vi "SUB_ContinueCom1Read.vi"(3 "error out 2":errorcluster, 4 "Numeric":i32, 5 "duplicate VISA resource name 2":refnum<visa-resource-name>) -> (0 "error out":errorcluster, 1 "String":string, 2 "duplicate VISA resource name":refnum<visa-resource-name>)   [LabVIEW 2011]
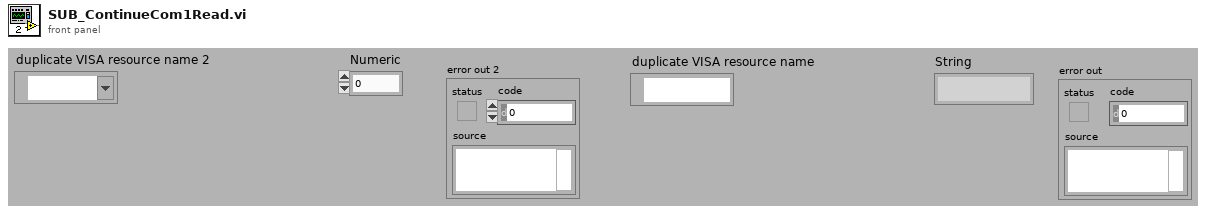
[diagram p1: front panel]
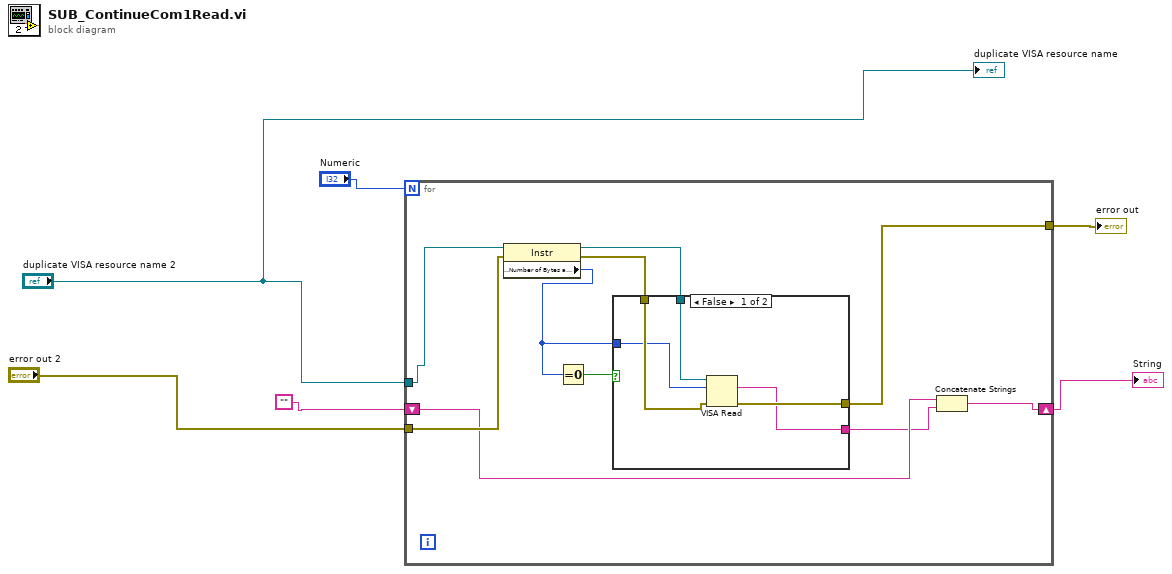
[diagram p0: block diagram]
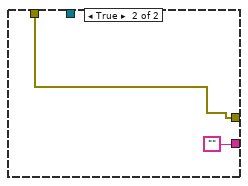
[diagram p2: hidden frame]
diagram:
  n1 = for {
    N: "Numeric" -> [_]
    shift-right: [w8] -> w6
    shift-left: "" -> [w9]
    tunnel: "duplicate VISA resource name 2" -> [w16]
    tunnel: "error out 2" -> [w15]
    tunnel: [w10] -> w1
    n2 = property on="Property Node" class="Instr"(reference=w16, error in=w15) -> (reference out=w11:refnum<visa-resource-name>, error out=w14:errorcluster, "Serial Settings:Number of Bytes at Serial Port"=w12:u32)
    n3 = Equal To 0?(x=w12) -> (x = 0?=w13:bool)
    n4 = case shown="False" w13 {
      tunnel: w14 -> [w21 w23]
      tunnel: w12 -> [w20 _]
      tunnel: w11 -> [w19 _]
      tunnel: [w18 w23] -> w10
      tunnel: [w17 ""] -> w7
      frame False {
        n5 = VISA Read(VISA resource name=w19, byte count=w20, error in (no error)=w21) -> (read buffer=w17:string, error out=w18:errorcluster)  [unwired: 2 out]
      }
      frame True {
      }
    }
    n6 = Concatenate Strings(w9, w7) -> (w8:string)
  }
  "error out" <- w1
  "String" <- w6
  "duplicate VISA resource name" <- "duplicate VISA resource name 2"
